vi "ObjectHandler.GetReference.vi"(8 "error in (no error)":errorcluster, 10 "Name":string, 11 "ObjectHandler in":refnum<class "ObjectHandler.lvclass">) -> (0 "error out":errorcluster, 1 "Found?":bool, 2 "ObjectWType":T1={"ObjectType"=enum."ObjectHandler", "Object"=variant}, 3 "ObjectHandler out":refnum<class "ObjectHandler.lvclass">)   [LabVIEW 2016, in "ObjectHandler.lvclass"]
uses:
  ObjectHandler.lvclass
  ObjectHandler.ObjectWType.ctl
  ObjectHandler.ObjectType.ctl
  ObjectHandler.lvclass/ObjectHandler.ctl
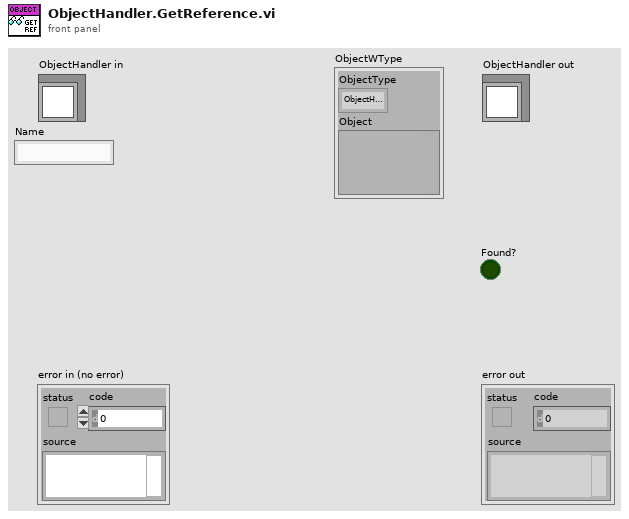
[diagram p1: front panel]
types:
  T1 = typedef "ObjectHandler.lvclass/ObjectHandler.ObjectWType.ctl" = cluster{"ObjectType":T2, "Object":variant}
  T2 = typedef "ObjectHandler.lvclass/ObjectHandler.ObjectType.ctl" = enum16{"undefined", "ObjectHandler", "ViHandler", "ErrorHandler", "CentralStorage", "Hausmodell", "Sondenmodell", "Wärmepumpe", "Umgebung"}
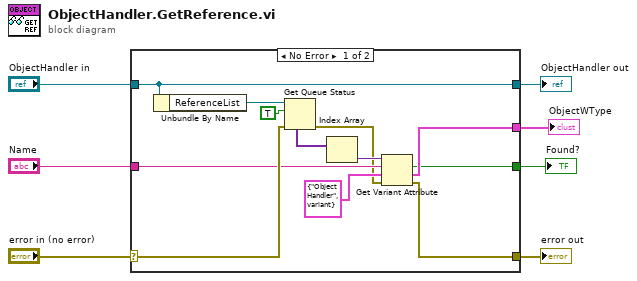
[diagram p0: block diagram]
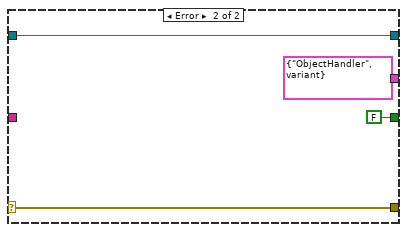
[diagram p2: hidden frame]
diagram:
  n1 = case shown="No Error" "error in (no error)" {
    selector: "error in (no error)" -> [w17 w22]
    tunnel: [w9 w22] -> w6
    tunnel: [w19 w23] -> w4
    tunnel: "ObjectHandler in" -> [w19 w23]
    tunnel: "Name" -> [w13 _]
    tunnel: [w11 T1 {"ObjectType"=enum."ObjectHandler", "Object"=variant} ("ObjectWType")] -> w2
    tunnel: [w8 FALSE] -> w1
    frame No Error {
      n2 = Unbundle By Name(w19) -> ("ReferenceList"=w18:refnum<queue>)
      n3 = Get Queue Status(queue=w18, return elements? (F)=TRUE, error in (no error)=w17) -> (error out=w10:errorcluster, elements=w16:variant[])  [unwired: 6 out]
      n4 = Index Array(array=w16) -> (element=w14:variant)  [unwired: 1 in]
      n5 = Get Variant Attribute(Variant=w14, name=w13, default value (empty Variant)=T1 {"ObjectType"=enum."ObjectHandler", "Object"=variant} ("ObjectWType"), error in=w10) -> (found=w8:bool, value=w11:T1, error out=w9:errorcluster)  [unwired: 1 out]
    }
    frame Error {
    }
  }
  "error out" <- w6
  "ObjectHandler out" <- w4
  "ObjectWType" <- w2
  "Found?" <- w1
